vi "ADS1015 Init.vi"(7 "I2C Channel":u8=1, 8 "error in (no error)":errorcluster, 9 "ADS1015 Config Options":T1={"Channel"=4, "Expected Range (Programmable Gain Amplifier)"=0, "Sampling Mode"=1, "Sampling Rate"=4, "Comparator Mode"=1, "Comparator Polarity"=1, "Latching Comparator"=1, "Comparator Queue & Disable"=3} {"Comparator Queue & Disable" items=["Assert after one conversion", "Assert after two conversions", "Assert after four conversions", "Comparator disabled"]; "Latching Comparator" items=["Non-latching", "Latching"]; "Comparator Polarity" items=["Active Low", "Active High"]; "Comparator Mode" items=["Traditional Comparator w/ hysteresis", "Window Comparator"]; "Sampling Rate" items=["128SPS", "250SPS", "490SPS", "920SPS", "1600SPS", "2400SPS", "3300SPS"]; "Sampling Mode" items=["Continuous Conversion", "Single-shot (Low Power)"]; "Expected Range (Programmable Gain Amplifier)" items=["+/-6.144V", "+/-4.096V", "+/-2.048V", "+/-1.024V", "+/-0.512V", "+/-0.256V"]; "Channel" items=["Differential: Ch 0&1", "Differential: Ch 0&3", "Differential: Ch 1&3", "Differential: Ch 2&3", "Single Ended: Ch 0", "Single Ended: Ch 1", "Single Ended: Ch 2", "Single Ended: Ch 3"]}, 10 "I2C Slave Address":u8=72 format="%.0x", 11 "LINX Resource in":T2) -> (0 "error out":errorcluster, 1 "ADS1015 Config Options":T1={"Channel"=4, "Expected Range (Programmable Gain Amplifier)"=0, "Sampling Mode"=1, "Sampling Rate"=4, "Comparator Mode"=1, "Comparator Polarity"=1, "Latching Comparator"=1, "Comparator Queue & Disable"=3} {"Comparator Queue & Disable" items=["Assert after one conversion", "Assert after two conversions", "Assert after four conversions", "Comparator disabled"]; "Latching Comparator" items=["Non-latching", "Latching"]; "Comparator Polarity" items=["Active Low", "Active High"]; "Comparator Mode" items=["Traditional Comparator w/ hysteresis", "Window Comparator"]; "Sampling Rate" items=["128SPS", "250SPS", "490SPS", "920SPS", "1600SPS", "2400SPS", "3300SPS"]; "Sampling Mode" items=["Continuous Conversion", "Single-shot (Low Power)"]; "Expected Range (Programmable Gain Amplifier)" items=["+/-6.144V", "+/-4.096V", "+/-2.048V", "+/-1.024V", "+/-0.512V", "+/-0.256V"]; "Channel" items=["Differential: Ch 0&1", "Differential: Ch 0&3", "Differential: Ch 1&3", "Differential: Ch 2&3", "Single Ended: Ch 0", "Single Ended: Ch 1", "Single Ended: Ch 2", "Single Ended: Ch 3"]}, 3 "LINX Resource out":T2)   [LabVIEW 2014]
uses:
  <vilib>/MakerHub/LINX/Private/Type Defs/LINX Ref.ctl
  <vilib>/MakerHub/LINX/Private/Type Defs/Platform.ctl
  <vilib>/MakerHub/LINX/Private/Type Defs/Interface.ctl
  <vilib>/MakerHub/LINX/Private/Device/Type Defs/LINX Device Config.ctl
  <vilib>/MakerHub/LINX/Private/Device/Type Defs/TCP Config.ctl
  <vilib>/MakerHub/LINX/Private/Device/Type Defs/Channels.ctl
  ADS1015 Config Options.ctl
  <vilib>/MakerHub/LINX/Private/Local IO/LinxI2cWrite.vi
  <vilib>/MakerHub/LINX/Public/Utilities/Check Channel.vi
  <vilib>/myRIO/Instrument Drivers/Onboard IO/I2C/vis/Write.vi
  <vilib>/MakerHub/LINX/Private/Utilties/Generate Error.vi
  <vilib>/MakerHub/LINX/Private/Utilties/Channel FGVs/I2C Channels.vi
  <vilib>/Utility/error.llb/Error Cluster From Error Code.vi
  <vilib>/myRIO/Common/Instrument Driver Framework/myRIO v1.0/I2C/vis/myRIO v1.0 Write I2C.vi
  <vilib>/MakerHub/LINX/LMH-LINX.lvlib
  <vilib>/MakerHub/LINX/Private/Device/Device.lvlib
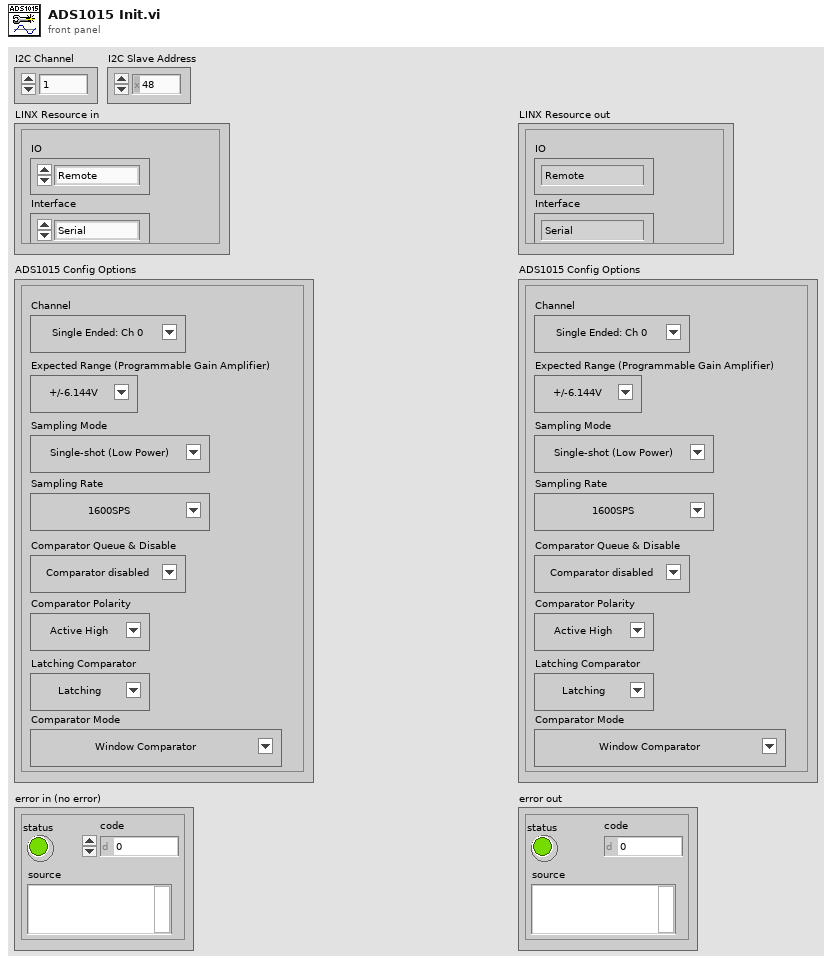
[diagram p1: front panel]
types:
  T1 = typedef "ADS1015 Config Options.ctl" = cluster{"Channel":u8, "Expected Range (Programmable Gain Amplifier)":u8, "Sampling Mode":u8, "Sampling Rate":u8, "Comparator Mode":u8, "Comparator Polarity":u8, "Latching Comparator":u8, "Comparator Queue & Disable":u8}
  T2 = typedef "LMH-LINX.lvlib/LINX Ref.ctl" = cluster{"IO":T3, "Interface":T4, "LINX Device Config":T5}
  T3 = typedef "LMH-LINX.lvlib/Platform.ctl" = enum16{"Remote", "Local"}
  T4 = typedef "LMH-LINX.lvlib/Interface.ctl" = enum16{"Serial", "TCP"}
  T5 = typedef "LMH-LINX.lvlib/Device.lvlib/LINX Device Config.ctl" = cluster{"Interface":T4, "COM Port":refnum<visa-resource-name>, "TCP Configuration":T6, "Device Family":u8, "Device ID":u8, "Device Name":string, "TCP Ref":refnum<k5>, "Channels":T7}
  T6 = typedef "LMH-LINX.lvlib/Device.lvlib/TCP Config.ctl" = cluster{"IP Address":string, "Port":u16}
  T7 = typedef "LMH-LINX.lvlib/Channels.ctl" = cluster{"DI":u8[], "DO":u8[], "AI":u8[], "AO":u8[], "PWM":u8[], "QE":u8[], "UART":u8[], "I2C 2":u8[], "SPI":u8[], "CAN":u8[], "Servo":u8[], "AI Ref (V)":dbl, "AI Resolution (Bits)":u8, "AO Ref (V)":dbl, "AO Resolution (Bits)":u8}
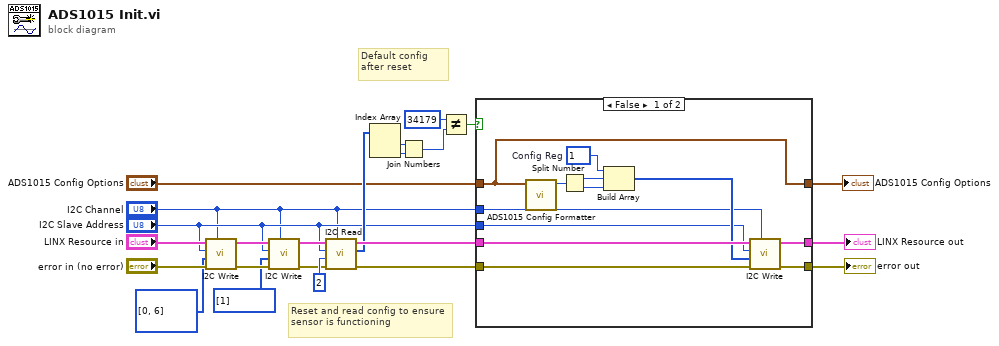
[diagram p0: block diagram]
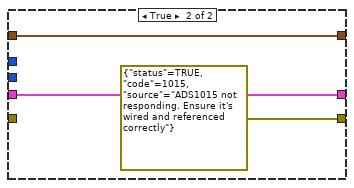
[diagram p2: hidden frame]
diagram:
  # "Default config after reset"
  # "Reset and read config to ensure sensor is functioning"
  n1 = call <vilib>:"I2C Write.vi"("I2C Channel"="I2C Channel", "Error In"="error in (no error)", "Data"=u8[] [0, 6], "I2C Slave Address (0)"="I2C Slave Address", "LINX Resource"="LINX Resource in") -> ("Error Out"=w9:errorcluster, "LINX Resource"=w8:T2)  [unwired: 5 in]
  n2 = call <vilib>:"I2C Write.vi"("I2C Channel"="I2C Channel", "Error In"=w9, "Data"=u8[] [1], "I2C Slave Address (0)"="I2C Slave Address", "LINX Resource"=w8) -> ("Error Out"=w6:errorcluster, "LINX Resource"=w7:T2)  [unwired: 5 in]
  n3 = call <vilib>:"I2C Read.vi"("I2C Channel"="I2C Channel", "Error In"=w6, "Bytes To Read"=u8 2, "I2C Slave Address (0)"="I2C Slave Address", "LINX Resource"=w7) -> ("Error Out"=w19:errorcluster, "Data"=w14:u8[], "LINX Resource"=w20:T2)  [unwired: 4 in]
  n4 = Index Array(array=w14) -> (element #1=w12:u8, element #2=w13:u8)  [unwired: 2 in]
  n5 = Join Numbers(hi=w12, lo=w13) -> ((hi.lo)=w11:u16)
  n6 = Not Equal?(x=u16 34179, y=w11) -> (x != y?=w15:bool)
  n7 = case shown="False" w15 {
    tunnel: w20 -> [w35 w38]
    tunnel: [w26 w38] -> w22
    tunnel: w19 -> [w34 _]
    tunnel: [w25 errorcluster {"status"=TRUE, "code"=1015, "source"="ADS1015 not responding. Ensure it's wired and referenced correctly"} ("error constant")] -> w21
    tunnel: "I2C Channel" -> [w28 _]
    tunnel: "I2C Slave Address" -> [w27 _]
    tunnel: "ADS1015 Config Options" -> [w24 w36]
    tunnel: [w24 w36] -> w1
    frame False {
      w30 = u8 1  # Config Reg
      n8 = call "ADS1015 Config Formatter.vi"("ADS1015 Config Options"=w24) -> ("Config Command"=w33:u16)  [unwired: 10 in]
      n9 = Split Number(x=w33) -> (hi(x)=w32:u8, lo(x)=w31:u8)
      n10 = Build Array(w30, w32, w31) -> (w29:u8[])
      n11 = call <vilib>:"I2C Write.vi"("I2C Channel"=w28, "Error In"=w34, "Data"=w29, "I2C Slave Address (0)"=w27, "LINX Resource"=w35) -> ("Error Out"=w25:errorcluster, "LINX Resource"=w26:T2)  [unwired: 5 in]
    }
    frame True {
    }
  }
  "error out" <- w21
  "LINX Resource out" <- w22
  "ADS1015 Config Options" <- w1
